vi "BarcodeprintR567.vi"() -> ()   [LabVIEW 2020]
uses:
  System.Drawing
  BarcodeLib.dll
  Sources/Global_Variable/Global.vi
panel:
  out "error out":errorcluster
  in  "错误输入（无错误）":errorcluster
  in  "保存位置":string="D:\\"
  in  "二维码颜色":u32(colorbox)
  in  "背景颜色":u32(colorbox)=16777215
  in  "单选按钮":enum32{"保存", "打印"}(radio)=enum."打印"
  in  "包含条形码标签":bool
  out "二维码图片":picture
  in  "高度":i32=200
  in  "宽度":i32=700
  in  "保存类型":i32(ring)=2 items=["JPG", "BMP", "PNG", "GIF", "TIFF", "UNSPECIFIED"]
  in  "编码类型":i32(ring)=27 items=["UNSPECIFIED", "UPCA", "UPCE", "UPC_SUPPLEMENTAL_2DIGIT", "UPC_SUPPLEMENTAL_5DIGIT", "EAN13", "EAN8", "Interleaved2of5", "Standard2of5", "Industrial2of5", "CODE39", "CODE39Extended", "Codabar", "PostNet", "BOOKLAND", "ISBN", "JAN13", "MSI_Mod10", "MSI_2Mod10", "MSI_Mod11", "MSI_Mod11_Mod10", "Modified_Plessey", "CODE11", "USD8", "UCC12", "UCC13", "LOGMARS", "CODE128", "CODE128A", "CODE128B", "CODE128C", "ITF14", "CODE93", "TELEPEN", "FIM"]
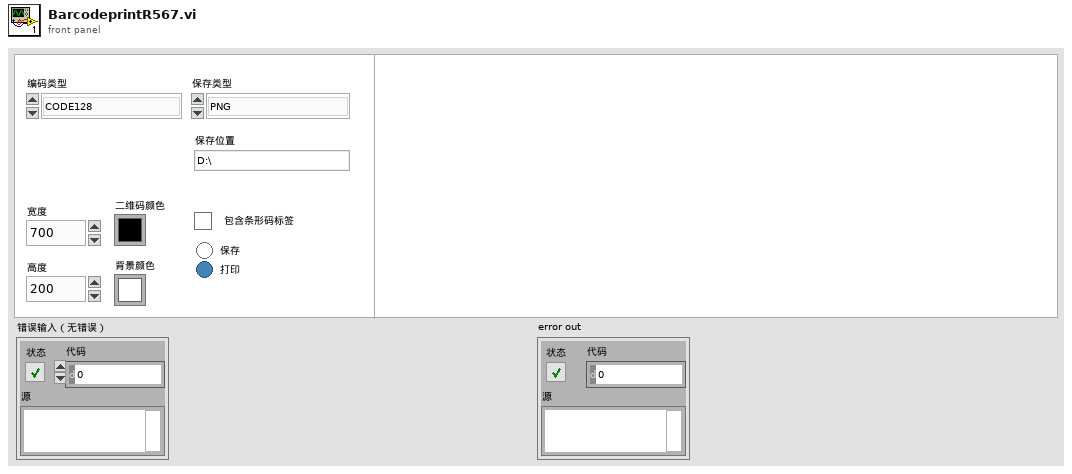
[diagram p1: front panel]
types:
  T1 = typedef "imagedata.ctl" = cluster{"image type":i32, "image depth":i32, "image":u8[], "mask":u8[], "colors":u32[], "Rectangle":cluster{"left":i16, "top":i16, "right":i16, "bottom":i16}}
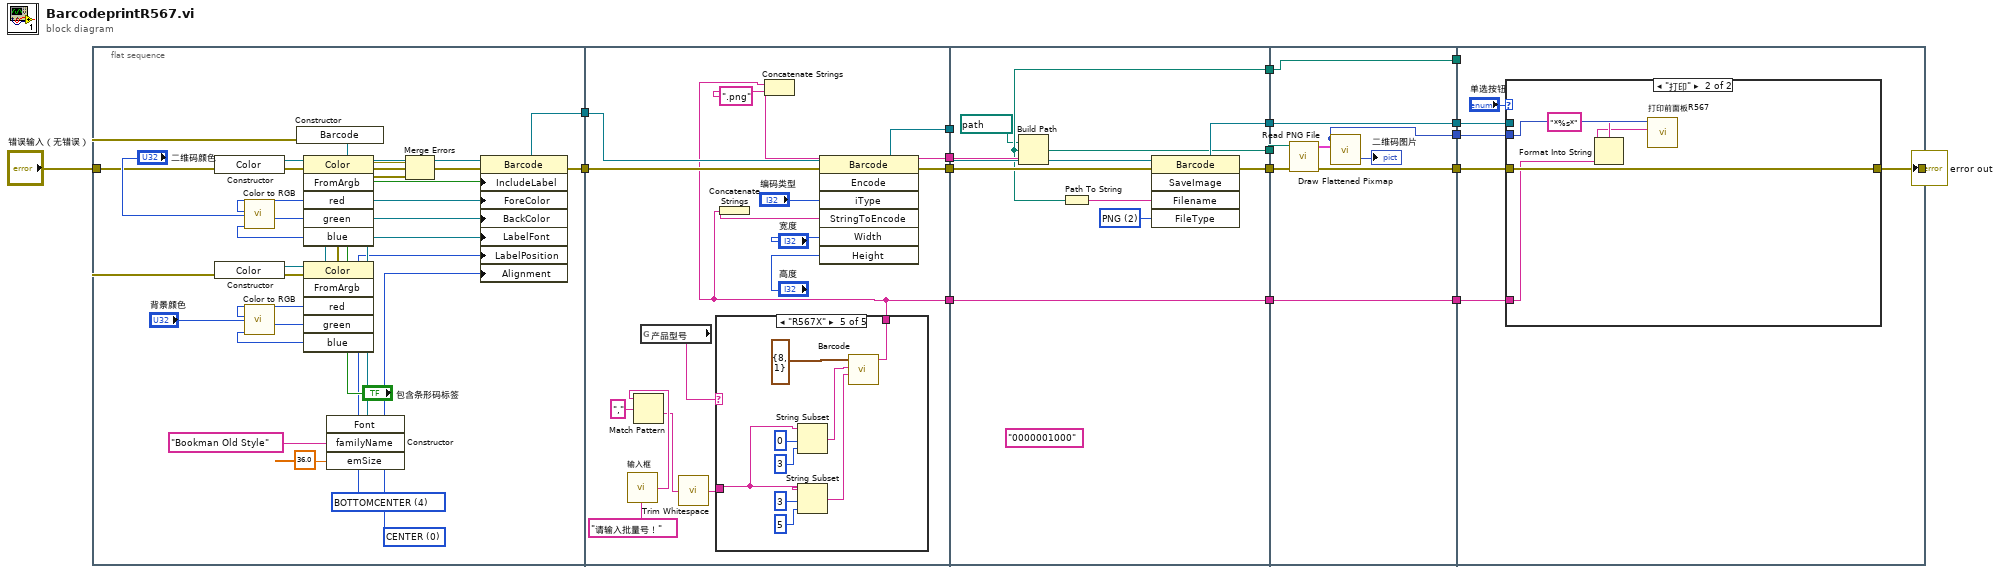
[diagram p0: block diagram]
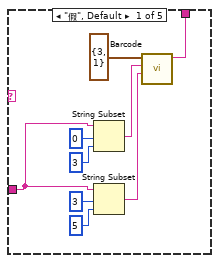
[diagram p2: hidden frame]
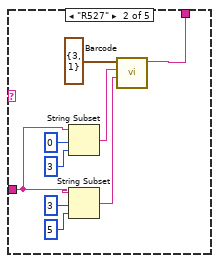
[diagram p3: hidden frame]
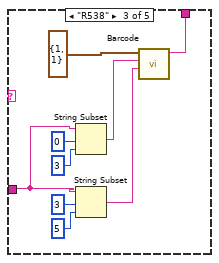
[diagram p4: hidden frame]
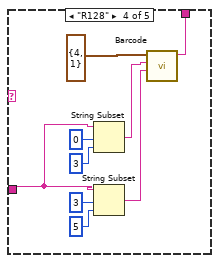
[diagram p5: hidden frame]
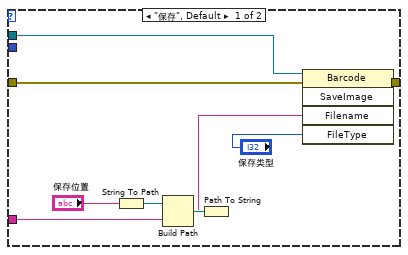
[diagram p6: hidden frame]
diagram:
  n1 = flat-sequence {
    tunnel: [w45] -> w18
    tunnel: [w44] -> w17
    tunnel: "错误输入（无错误）" -> [w24]
    tunnel: w18 -> [w62]
    tunnel: w17 -> [w61]
    tunnel: [w60] -> w16
    tunnel: [w59] -> w15
    tunnel: [w57] -> w14
    tunnel: [w53] -> w1
    tunnel: w16 -> [w118]
    tunnel: w15 -> [w117]
    tunnel: w14 -> [w113]
    tunnel: [w115] -> w13
    tunnel: [w114] -> w12
    tunnel: [w111] -> w11
    tunnel: [w109] -> w7
    tunnel: [w111] -> w5
    tunnel: w1 -> [w109]
    tunnel: w13 -> [w126]
    tunnel: w12 -> [w121]
    tunnel: w11 -> [w124]
    tunnel: [w126] -> w10
    tunnel: [w120] -> w9
    tunnel: [w123] -> w8
    tunnel: w7 -> [w123]
    tunnel: [w122] -> w6
    tunnel: w5 -> [w122]
    tunnel: [w119] -> w2
    tunnel: w10 -> [w131]
    tunnel: w9 -> [w130]
    tunnel: w8 -> [w129]
    tunnel: w6 -> [_]
    tunnel: [w128] -> w3
    tunnel: w2 -> [w127]
    frame #0 {
      w19 = 0 items=["CENTER", "LEFT", "RIGHT"] ("Alignment")
      w20 = 4 items=["TOPLEFT", "TOPCENTER", "TOPRIGHT", "BOTTOMLEFT", "BOTTOMCENTER", "BOTTOMRIGHT"] ("LabelPosition")
      n2 = constructor class="Color"(error in=w24) -> (reference out=w38:refnum<k24>, error out=w30:errorcluster)  [unwired: 2 in, 1 out]
      n3 = constructor class="Color"(error in=w24) -> (reference out=w36:refnum<k24>, error out=w29:errorcluster)  [unwired: 2 in, 1 out]
      n4 = call <vilib>:"Color to RGB.vi"("Color"="二维码颜色") -> ("R"=w41:u8, "G"=w40:u8, "B"=w39:u8)  [unwired: 1 out]
      n5 = call <vilib>:"Color to RGB.vi"("Color"="背景颜色") -> ("R"=w33:u8, "G"=w34:u8, "B"=w35:u8)  [unwired: 1 out]
      n6 = constructor class="Barcode"(error in=w24) -> (reference out=w46:refnum<k24>, error out=w27:errorcluster)  [unwired: 2 in, 1 out]
      n7 = invoke class="Color" method="FromArgb"(reference=w38, error in=w30, "red"=w41, "green"=w40, "blue"=w39) -> (error out=w28:errorcluster, "FromArgb"=w37:refnum<k24>)  [unwired: 1 in, 4 out]
      n8 = invoke class="Color" method="FromArgb"(reference=w36, error in=w29, "red"=w33, "green"=w34, "blue"=w35) -> (error out=w26:errorcluster, "FromArgb"=w32:refnum<k24>)  [unwired: 1 in, 4 out]
      n9 = constructor class="Font"("familyName"="Bookman Old Style", "emSize"=sgl 36.0) -> (reference out=w21:refnum<k24>)  [unwired: 3 in, 4 out]
      n10 = Merge Errors(w27, w28, w26) -> (w25:errorcluster)
      n11 = property on="属性节点" class="Barcode"(reference=w46, error in=w25, "IncludeLabel"="包含条形码标签", "ForeColor"=w37, "BackColor"=w32, "LabelFont"=w21, "LabelPosition"=w20, "Alignment"=w19) -> (reference out=w45:refnum<k24>, error out=w44:errorcluster)
    }
    frame #1 {
      n12 = call "输入框.vi"("提示信息"="请输入批量号！") -> ("条形码输出"=w48:string)
      n13 = Match Pattern(string=w48, regular expression="," ("正则表达式")) -> (after substring=w47:string)  [unwired: 1 in, 3 out]
      n14 = global read "Global.vi" "产品型号"() -> (w52:string)
      n15 = call <vilib>:"Trim Whitespace.vi"("string"=w47) -> ("trimmed string"=w50:string)  [unwired: 1 in]
      n16 = case shown="\"R567X\"" w52 {
        tunnel: [w66 w81 w89 w98 w107] -> w53
        tunnel: w50 -> [w64 w75 w84 w93 w102]
        frame "假", Default {
          n17 = String Subset(string=w64, offset (0)=0 ("偏移量(0)"), length (rest)=3 ("长度（剩余）")) -> (substring=w72:string)
          n18 = String Subset(string=w64, offset (0)=3 ("偏移量(0)"), length (rest)=5 ("长度（剩余）")) -> (substring=w71:string)
          n19 = call "Barcode.vi"("流水号"=w71, "年月日"=w72, "start (0, 0)"=cluster{"start row":i32, "start column":i32} {"start row"=3, "start column"=1}) -> ("条形码"=w66:string)  [unwired: 8 in]
        }
        frame "R527" {
          n20 = String Subset(string=w75, offset (0)=0 ("偏移量(0)"), length (rest)=3 ("长度（剩余）")) -> (substring=w74:string)
          n21 = String Subset(string=w75, offset (0)=3 ("偏移量(0)"), length (rest)=5 ("长度（剩余）")) -> (substring=w73:string)
          n22 = call "Barcode.vi"("流水号"=w73, "年月日"=w74, "start (0, 0)"=cluster{"start row":i32, "start column":i32} {"start row"=3, "start column"=1}) -> ("条形码"=w81:string)  [unwired: 8 in]
        }
        frame "R538" {
          n23 = String Subset(string=w84, offset (0)=0 ("偏移量(0)"), length (rest)=3 ("长度（剩余）")) -> (substring=w83:string)
          n24 = String Subset(string=w84, offset (0)=3 ("偏移量(0)"), length (rest)=5 ("长度（剩余）")) -> (substring=w82:string)
          n25 = call "Barcode.vi"("流水号"=w82, "年月日"=w83, "start (0, 0)"=cluster{"start row":i32, "start column":i32} {"start row"=1, "start column"=1}) -> ("条形码"=w89:string)  [unwired: 8 in]
        }
        frame "R128" {
          n26 = String Subset(string=w93, offset (0)=0 ("偏移量(0)"), length (rest)=3 ("长度（剩余）")) -> (substring=w92:string)
          n27 = String Subset(string=w93, offset (0)=3 ("偏移量(0)"), length (rest)=5 ("长度（剩余）")) -> (substring=w91:string)
          n28 = call "Barcode.vi"("流水号"=w91, "年月日"=w92, "start (0, 0)"=cluster{"start row":i32, "start column":i32} {"start row"=4, "start column"=1}) -> ("条形码"=w98:string)  [unwired: 8 in]
        }
        frame "R567X" {
          n29 = String Subset(string=w102, offset (0)=0 ("偏移量(0)"), length (rest)=3 ("长度（剩余）")) -> (substring=w101:string)
          n30 = String Subset(string=w102, offset (0)=3 ("偏移量(0)"), length (rest)=5 ("长度（剩余）")) -> (substring=w100:string)
          n31 = call "Barcode.vi"("流水号"=w100, "年月日"=w101, "start (0, 0)"=cluster{"start row":i32, "start column":i32} {"start row"=8, "start column"=1}) -> ("条形码"=w107:string)  [unwired: 8 in]
        }
      }
      n32 = Concatenate Strings(w53) -> (w54:string)
      n33 = Concatenate Strings(w53, ".png" ("字符串")) -> (w57:string)
      n34 = invoke class="Barcode" method="Encode"(reference=w62, error in=w61, "iType"="编码类型", "StringToEncode"=w54, "Width"="宽度", "Height"="高度") -> (reference out=w60:refnum<k24>, error out=w59:errorcluster)  [unwired: 1 in, 5 out]
    }
    frame #2 {
      (unwired) "0000001000" ("条形码")
      w116 = 2 items=["JPG", "BMP", "PNG", "GIF", "TIFF", "UNSPECIFIED"] ("FileType")
      n35 = Build Path(base path=path "D:/条码" ("基路径"), name or relative path=w113) -> (appended path=w111:path)
      n36 = Path To String(path=w111) -> (string=w112:string)
      n37 = invoke class="Barcode" method="SaveImage"(reference=w118, error in=w117, "Filename"=w112, "FileType"=w116) -> (reference out=w115:refnum<k24>, error out=w114:errorcluster)  [unwired: 1 in, 3 out]
    }
    frame #3 {
      n38 = call <vilib>:"Read PNG File.vi"("error in (no error)"=w121, "path to PNG file"=w124) -> ("error out"=w120:errorcluster, "image data"=w125:T1)  [unwired: 7 in, 1 out]
      n39 = call <vilib>:"Draw Flattened Pixmap.vi"("image data"=w125) -> ("new picture"=w119:picture)  [unwired: 8 in]
      "二维码图片" <- w119
    }
    frame #4 {
      n40 = case shown="\"打印\"" "单选按钮" {
        tunnel: w131 -> [w141 _]
        tunnel: w130 -> [w140 w145]
        tunnel: w129 -> [w134 w143]
        tunnel: [w133 w145] -> w128
        tunnel: w127 -> [_ w146]
        frame "保存", Default {
          n41 = String To Path(string="保存位置") -> (path=w138:path)
          n42 = Build Path(base path=w138, name or relative path=w134) -> (appended path=w139:path)
          n43 = Path To String(path=w139) -> (string=w136:string)
          n44 = invoke class="Barcode" method="SaveImage"(reference=w141, error in=w140, "Filename"=w136, "FileType"="保存类型") -> (error out=w133:errorcluster)  [unwired: 1 in, 4 out]
        }
        frame "打印" {
          n45 = Format Into String(format string="*%s*" ("格式字符串"), w143) -> (resulting string=w142:string)  [unwired: 2 in, 1 out]
          n46 = call "打印前面板R567.vi"("字符串"=w142, "二维码图片"=w146) -> ()  [unwired: 10 in]
        }
      }
    }
  }
  "error out" <- w3
